vi "cursors settings.vi"(5 "Cursor color":u32(colorbox), 7 "Starting cursor":i32, 8 "error in (no error)":errorcluster, 9 "Show cursors":bool, 10 "App Data":T1, 11 "XYGraph in":refnum<vi>) -> (0 "error out":errorcluster)   [LabVIEW 2014]
uses:
  Controls/App Data.ctl
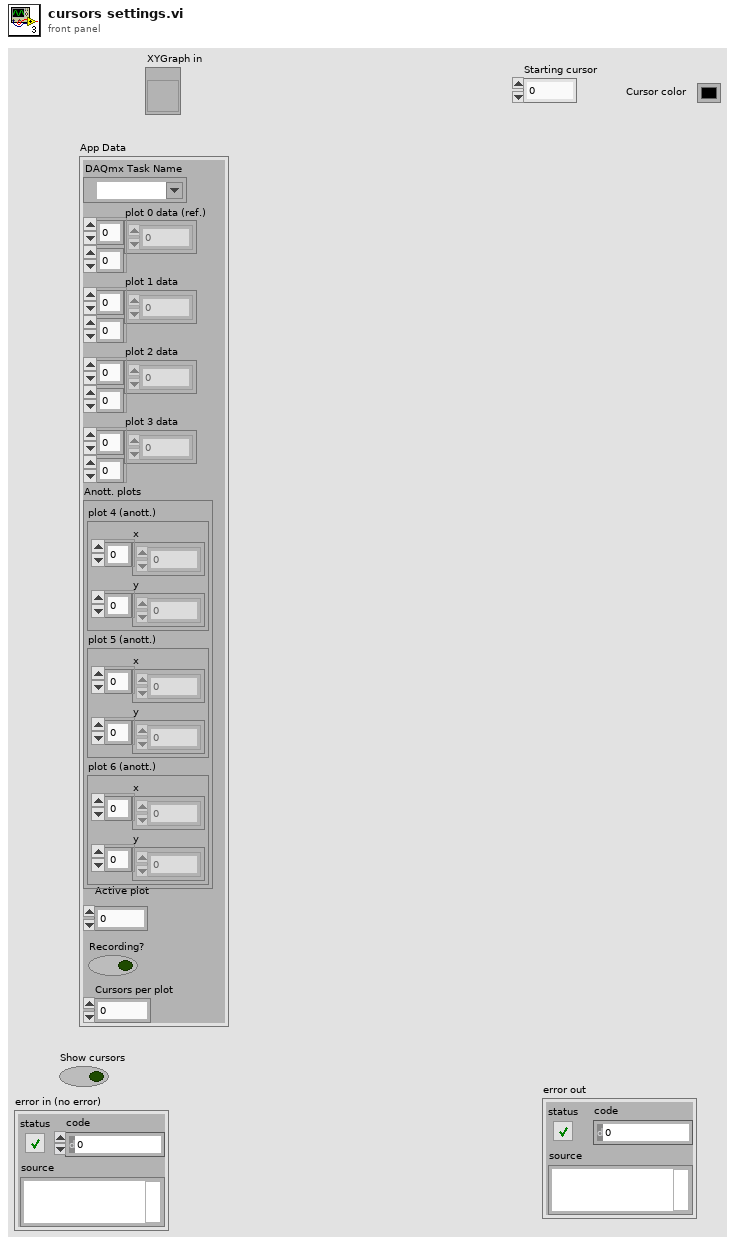
[diagram p1: front panel]
types:
  T1 = typedef "App Data.ctl" = cluster{"DAQmx Task Name":refnum<k21>, "plot 0 data (ref.)":dbl[][], "plot 1 data":dbl[][], "plot 2 data":dbl[][], "plot 3 data":dbl[][], "Anott. plots":cluster{"plot 4 (anott.)":cluster{"x":dbl[], "y":dbl[]}, "plot 5 (anott.)":cluster{"x":dbl[], "y":dbl[]}, "plot 6 (anott.)":cluster{"x":dbl[], "y":dbl[]}}, "Active plot":u32, "Recording?":bool, "Cursors per plot":i32}
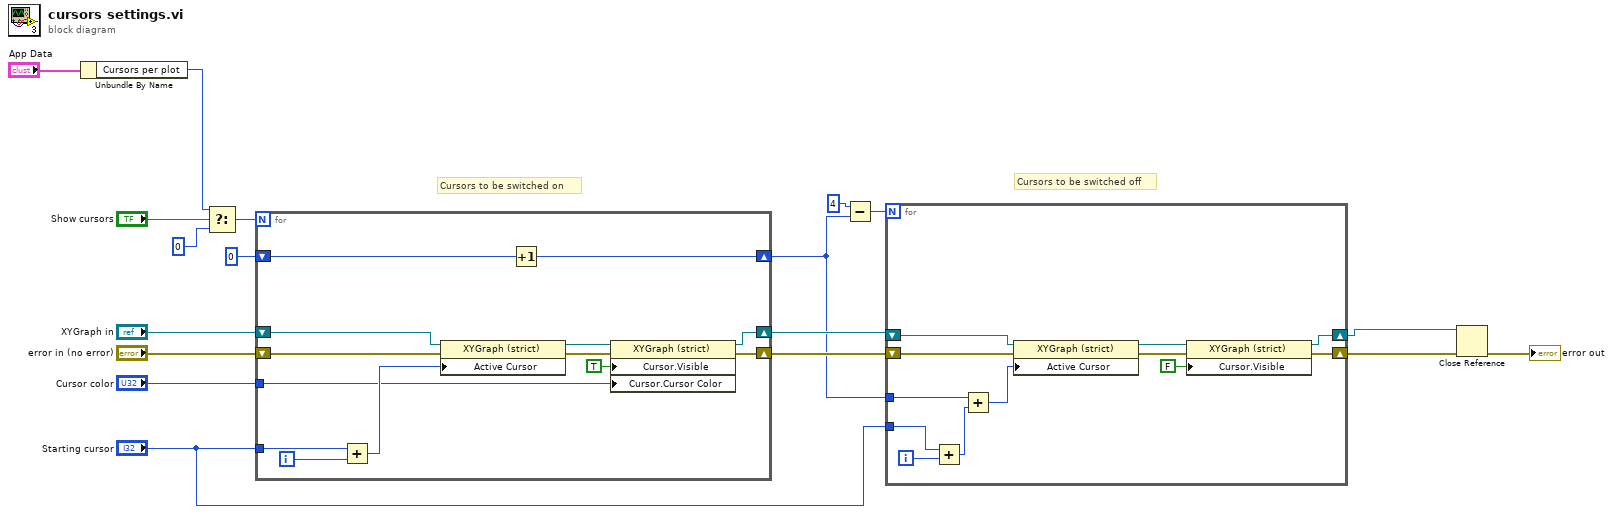
[diagram p0: block diagram]
diagram:
  # "Cursors to be switched off"
  # "Cursors to be switched on"
  n1 = Unbundle By Name("App Data") -> ("Cursors per plot"=w11:i32)
  n2 = Select(t=w11, s="Show cursors", f=0) -> (s? t:f=w10:i32)
  n3 = for {
    N: w10 -> [_]
    shift-right: [w29] -> w16
    shift-left: "error in (no error)" -> [w31]
    tunnel: "Starting cursor" -> [w24]
    shift-right: [w22] -> w8
    shift-left: "XYGraph in" -> [w26]
    shift-right: [w20] -> w2
    shift-left: 0 ("f") -> [w21]
    tunnel: "Cursor color" -> [w19]
    i -> [w28]
    n4 = Add(x=w24, y=w28) -> (x+y=w27:i32)
    n5 = property on="Property Node" class="XYGraph (strict)"(reference=w26, error in=w31, "Active Cursor"=w27) -> (reference out=w25:refnum<vi>, error out=w30:errorcluster)
    n6 = Increment(x=w21) -> (x+1=w20:i32)
    n7 = property on="Property Node" class="XYGraph (strict)"(reference=w25, error in=w30, "Cursor.Visible"=TRUE, "Cursor.Cursor Color"=w19) -> (reference out=w22:refnum<vi>, error out=w29:errorcluster)
  }
  n8 = Subtract(x=4, y=w2) -> (x-y=w17:i32)
  n9 = for {
    N: w17 -> [_]
    shift-right: [w39] -> w6
    shift-left: w16 -> [w42]
    shift-right: [w36] -> w7
    shift-left: w8 -> [w38]
    tunnel: "Starting cursor" -> [w35]
    tunnel: w2 -> [w32]
    i -> [w40]
    n10 = Add(x=w35, y=w40) -> (x+y=w34:i32)
    n11 = Add(x=w32, y=w34) -> (x+y=w33:i32)
    n12 = property on="Property Node" class="XYGraph (strict)"(reference=w38, error in=w42, "Active Cursor"=w33) -> (reference out=w37:refnum<vi>, error out=w43:errorcluster)
    n13 = property on="Property Node" class="XYGraph (strict)"(reference=w37, error in=w43, "Cursor.Visible"=FALSE) -> (reference out=w36:refnum<vi>, error out=w39:errorcluster)
  }
  n14 = Close Reference(reference=w7, error in (no error)=w6) -> (error out=→"error out":errorcluster)
